vi "ErrorDefinitionSQLite_LibraryInUseTest.vi"() -> ()   [LabVIEW 2018]
uses:
  ErrorDefinitionSQLite.lvclass
panel:
  out "SpecificErrorInUse":bool
  out "FreeErrorsInLibrary":i32
  out "LibraryInUse":bool
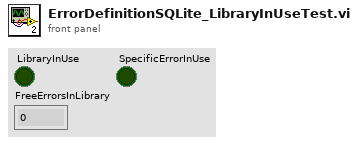
[diagram p1: front panel]
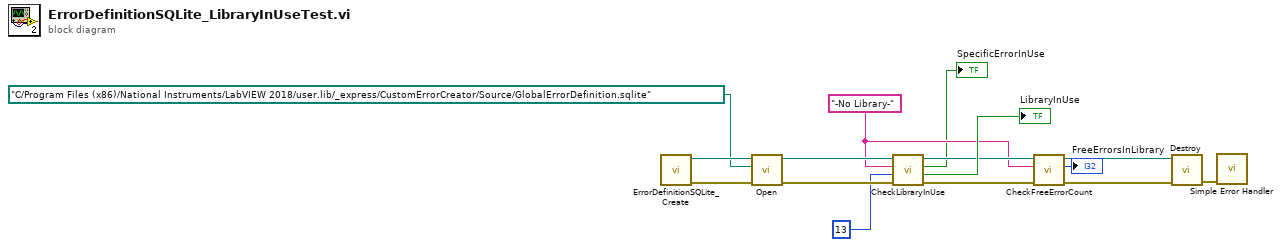
[diagram p0: block diagram]
diagram:
  w3 = "-No Library-" ("Library")
  n1 = call "ErrorDefinitionSQLite_Create.vi"() -> ("ErrorOut"=w14:errorcluster, "Reference out"=w15:refnum<class "ErrorDefinitionSQLite.lvclass">)  [unwired: 10 in]
  n2 = call-dynamic "Open.vi"("ErrorIn"=w14, "Path"=path "C:/Program Files (x86)/National Instruments/LabVIEW 2018/user.lib/_express/CustomErrorCreator/Source/GlobalErrorDefinition.sqlite", "ReferenceIn"=w15) -> ("ErrorOut"=w10:errorcluster, "ReferenceOut"=w11:refnum<class "ErrorDefinitionSQLite.lvclass">)  [unwired: 7 in]
  n3 = call-dynamic "CheckLibraryInUse.vi"("ErrorIn"=w10, "ErrorCode"=13, "Library"=w3, "ReferenceIn"=w11) -> ("ErrorOut"=w7:errorcluster, "LibraryInUse"=→"LibraryInUse":bool, "SpecificErrorInUse"=→"SpecificErrorInUse":bool, "ReferenceOut"=w6:refnum<class "ErrorDefinitionSQLite.lvclass">)  [unwired: 4 in]
  n4 = call-dynamic "CheckFreeErrorCount.vi"("ErrorIn"=w7, "Library"=w3, "ReferenceIn"=w6) -> ("ErrorOut"=w4:errorcluster, "FreeErrorsInLibrary"=→"FreeErrorsInLibrary":i32, "ReferenceOut"=w5:refnum<class "ErrorDefinitionSQLite.lvclass">)  [unwired: 6 in]
  n5 = call-dynamic "Destroy.vi"("ErrorIn"=w4, "Reference in"=w5) -> ("ErrorOut"=w12:errorcluster)  [unwired: 8 in, 1 out]
  n6 = call <vilib>:"Simple Error Handler.vi"("error in (no error)"=w12) -> ()  [unwired: 4 in, 5 out]
